vi "Scale Plots.vi"(0 "Data in":T6, 5 "Display State":T1, 9 "panel":refnum<vi>) -> (15 "error out":errorcluster)   [LabVIEW 2015, in "Interactive Graph.xctl"]
uses:
  Interactive Graph.xctl
  Data.vi
  EPhys/LV Source/Work Panel VIs/Typedefs/EPhysWork-Label Position.ctl
  State.vi
  Persistent.ctl
  Plot.ctl
  Events.ctl
  Selection.ctl
  XRange.ctl
  YScale.ctl
  Cursor.ctl
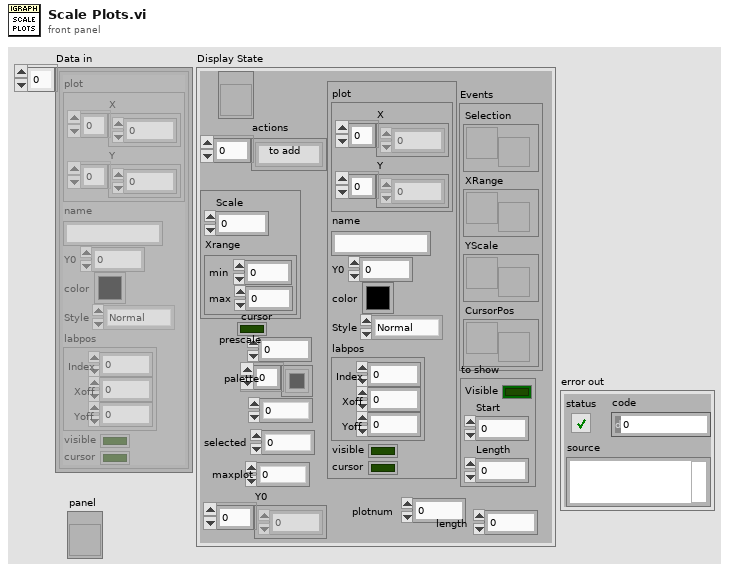
[diagram p1: front panel]
types:
  T1 = typedef "Interactive Graph.xctl/State.vi" = cluster{"ref":refnum<vi>, "actions":string[], "Persist":T2, "cursor":bool, "prescale":dbl, "palette":u32[], "colIndex":i32, "to add":T3, "Events":T5, "selected":i32, "to show":cluster{"Visible":bool, "Start":i32, "Length":i32}, "maxplot":i32, "Y0":dbl[], "plotnum":i32, "length":i32}
  T2 = typedef "Interactive Graph.xctl/Persistent.ctl" = cluster{"Scale":dbl, "Xrange":cluster{"min":dbl, "max":dbl}}
  T3 = typedef "Interactive Graph.xctl/Plot.ctl" = cluster{"plot":cluster{"X":dbl[], "Y":dbl[]}, "name":string, "Y0":dbl, "color":u32, "Style":enum16{"Normal", "Highlight", "Shadow"}, "labpos":T4, "visible":bool, "cursor":bool}
  T4 = typedef "EPhysWork-Label Position.ctl" = cluster{"Index":i32, "Xoff":dbl, "Yoff":dbl}
  T5 = typedef "Interactive Graph.xctl/Events.ctl" = cluster{"Selection":refnum<user-event>, "XRange":refnum<user-event>, "YScale":refnum<user-event>, "CursorPos":refnum<user-event>}
  T6 = typedef "Interactive Graph.xctl/Data.vi" = cluster{"plot":cluster{"X":dbl[], "Y":dbl[]}, "name":string, "Y0":dbl, "color":u32, "Style":enum16{"Normal", "Highlight", "Shadow"}, "labpos":T4, "visible":bool, "cursor":bool}[]
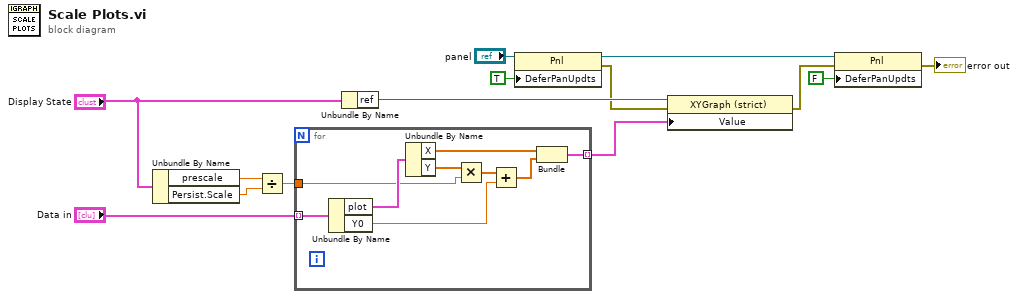
[diagram p0: block diagram]
diagram:
  n1 = Unbundle By Name("Display State") -> ("prescale"=w3:dbl, "Persist.Scale"=w2:dbl)
  n2 = Divide(x=w3, y=w2) -> (x/y=w1:dbl)
  n3 = for {
    tunnel: "Data in" -> [w15] mode=indexing
    tunnel: [w20] -> w12 mode=indexing
    tunnel: w1 -> [w21]
    n4 = Unbundle By Name(w15) -> ("plot"=w23:cluster{"X":dbl[], "Y":dbl[]}, "Y0"=w17:dbl)
    n5 = Unbundle By Name(w23) -> ("X"=w16:dbl[], "Y"=w22:dbl[])
    n6 = Multiply(x=w22, y=w21) -> (x*y=w18:dbl[])
    n7 = Add(x=w18, y=w17) -> (x+y=w19:dbl[])
    n8 = Bundle("X"=w16, w19) -> (w20:cluster{"X":dbl[], dbl[]})  [unwired: 1 in]
  }
  n9 = Unbundle By Name("Display State") -> ("ref"=w13:refnum<vi>)
  n10 = property class="Pnl"(reference="panel", "DeferPanUpdts"=TRUE ("Defer Panel Updates")) -> (reference out=w6:refnum<vi>, error out=w10:errorcluster)  [unwired: 1 in]
  n11 = property class="XYGraph (strict)"(reference=w13, error in=w10, "Value"=w12) -> (error out=w11:errorcluster)  [unwired: 1 out]
  n12 = property class="Pnl"(reference=w6, error in=w11, "DeferPanUpdts"=FALSE ("Defer Panel Updates")) -> (error out=→"error out":errorcluster)  [unwired: 1 out]
